vi "gateway发消息.vi"() -> ()   [LabVIEW 2012]
uses:
  <vilib>/LabVIEW Targets/Embedded/WSN/Host API/WSN Msg Status.ctl
panel:
  out "message status":T1
  in  "停止":bool
  in  "更改":bool
  in  "取消按钮":bool
  out "节点信息":string
  in  "节点":i32(listbox)
  in  "确定按钮":bool
  out "返回消息":string
  in  "发消息":string
  in  "网关IP地址":string
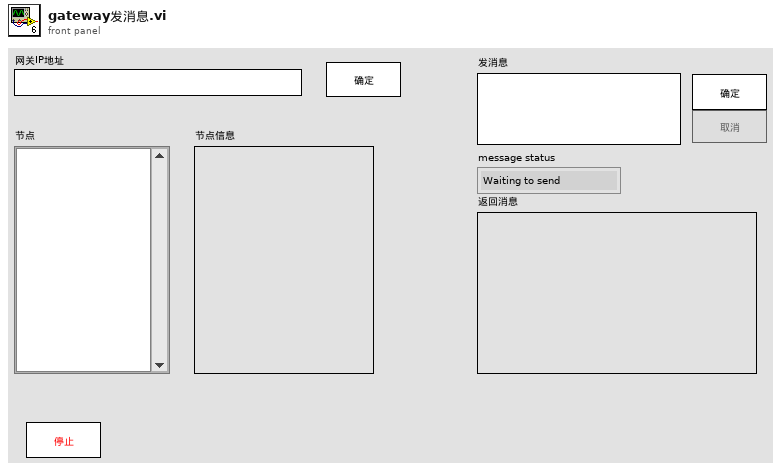
[diagram p1: front panel]
types:
  T1 = typedef "WSN Msg Status.ctl" = enum8{"Waiting to send", "Sent to node", "Failed", "Cancelled"}
  T2 = enum8{"Enabled", "Disabled", "Disabled and Grayed Out"}
  T3 = typedef "WSN Node Info.ctl" = cluster{"Serial Number":u32, "ID":u32, "Node Type":u16, "Firmware Update State":enum8{"Not Started", "In Progress", "Error", "Done"}, "Firmware Update Percent Complete":u8, "Current Firmware Version":string, "Battery State":u8, "Last Packet Received":timestamp, "Link Quality":enum16{"No Signal", "Poor", "Fair", "Good", "Excellent"}, "Power Supply":enum8{"Battery", "Externally Powered"}, "Network Mode":enum8{"End Device", "Mesh Router"}}
  T4 = typedef "WSN Message.ctl" = cluster{"Message Type":enum16{"User Message", "Debug Message"}, "Message Timestamp":timestamp, "Data":string}
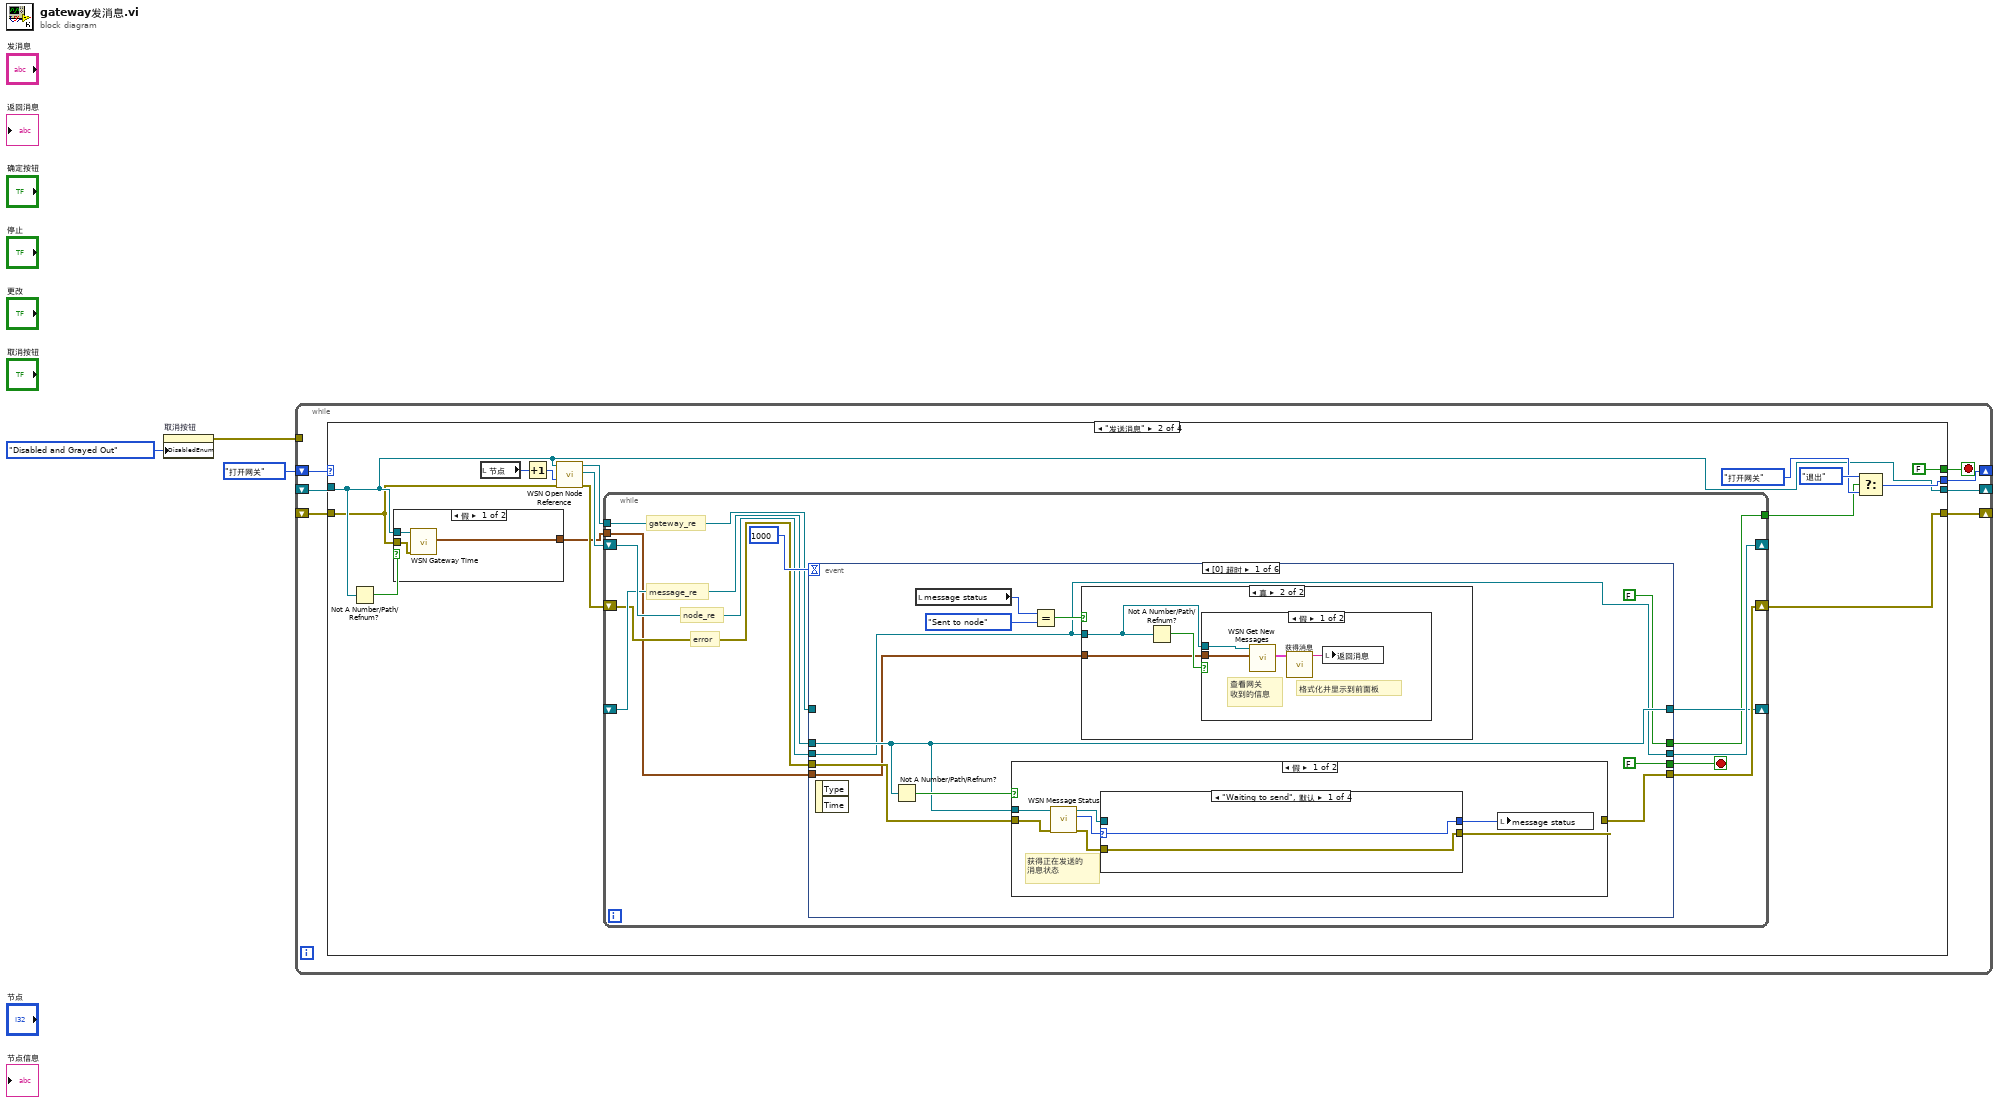
[diagram p0: block diagram]
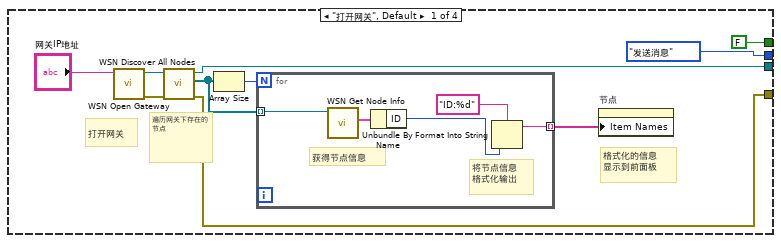
[diagram p2: hidden frame]
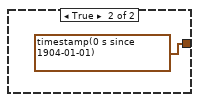
[diagram p3: hidden frame]
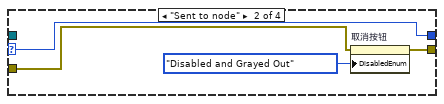
[diagram p6: hidden frame]
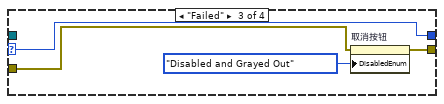
[diagram p7: hidden frame]
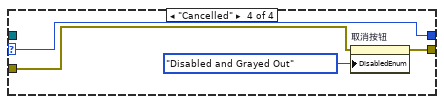
[diagram p8: hidden frame]
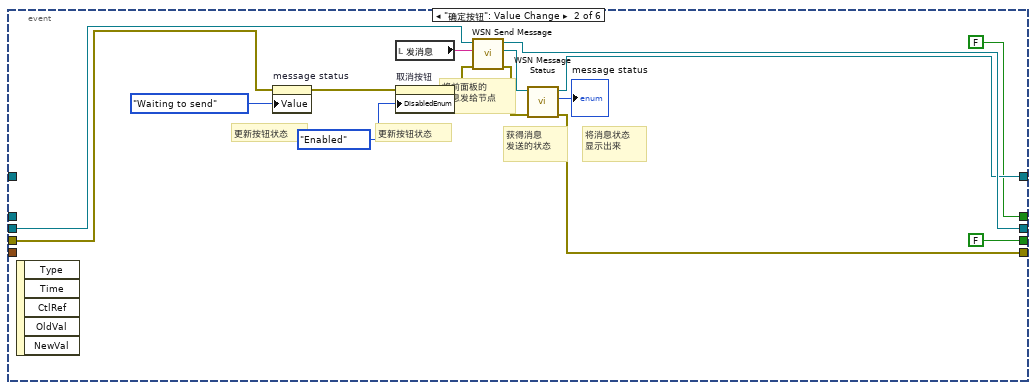
[diagram p10: hidden frame]
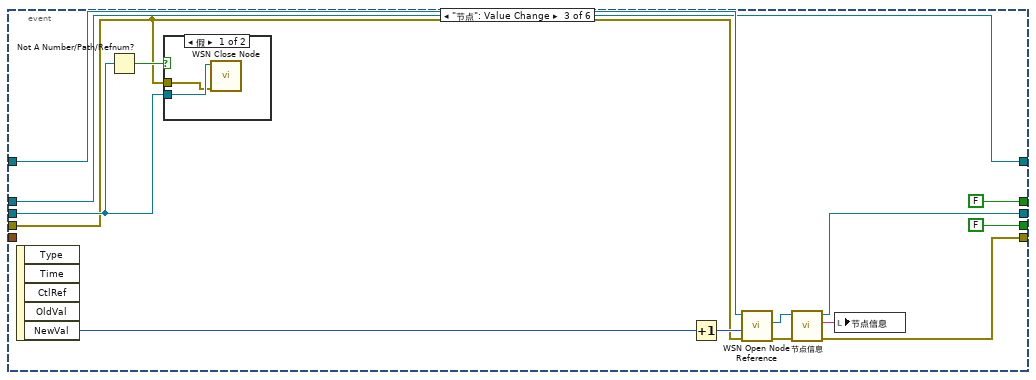
[diagram p11: hidden frame]
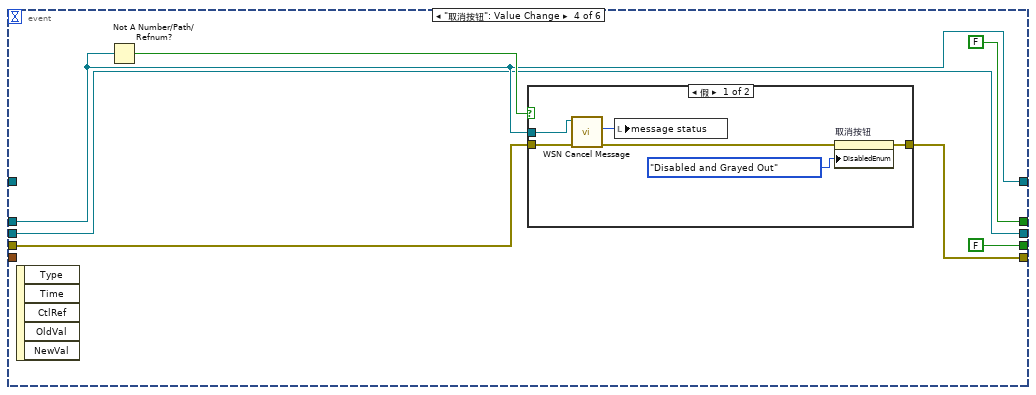
[diagram p13: hidden frame]
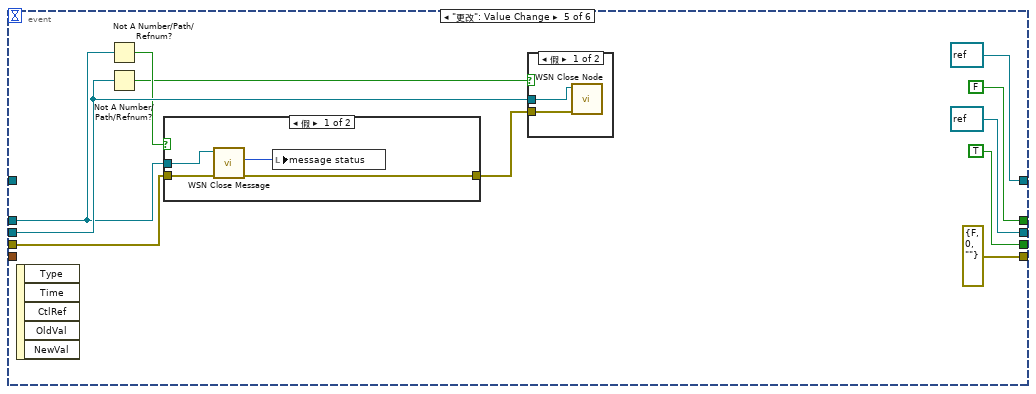
[diagram p15: hidden frame]
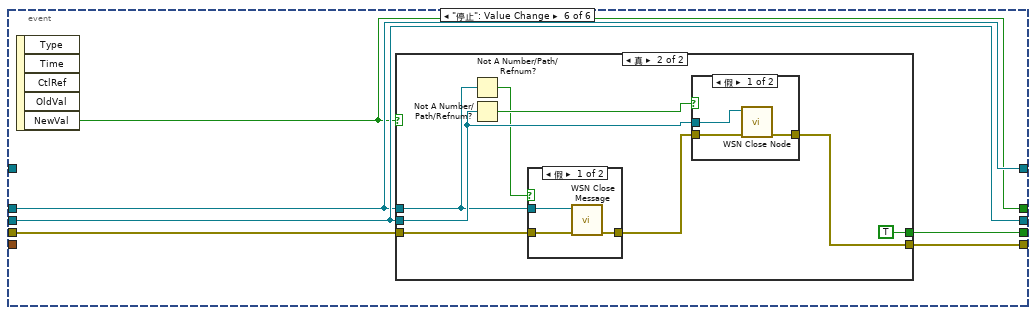
[diagram p18: hidden frame]
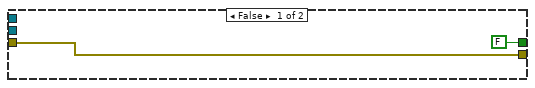
[diagram p19: hidden frame]
diagram:
  n1 = property on="取消按钮" class="Bool"("DisabledEnum"=T2."Disabled and Grayed Out" ("禁用")) -> (error out=w1:errorcluster)  [unwired: 2 in, 1 out]
  n2 = while {
    shift-right: [w4] -> _
    shift-left: enum16{"打开网关", "发送消息", "关闭网关", "退出"}."打开网关" -> [w10]
    shift-right: [w9] -> _
    shift-left: _ -> [w7]
    shift-right: [w8] -> _
    shift-left: _ -> [w6]
    tunnel: w1 -> [_]
    stop <- w5 stop-if-true
    n3 = case shown="\"发送消息\"" w10 {
      tunnel: [w14 w28 w184 refnum<k20> refnum ("gateway reference")] -> w9
      tunnel: [w13 w37 errorcluster {"status"=FALSE, "code"=0, "source"=""} ("error out") errorcluster {"status"=FALSE, "code"=0, "source"=""} ("error out")] -> w8
      tunnel: w7 -> [_ w28 w184 w192]
      tunnel: w6 -> [_ w27 w188 w196]
      tunnel: [FALSE FALSE FALSE TRUE] -> w5
      tunnel: [enum16{"打开网关", "发送消息", "关闭网关", "退出"}."发送消息" w35 enum16{"打开网关", "发送消息", "关闭网关", "退出"}."打开网关" enum16{"打开网关", "发送消息", "关闭网关", "退出"}."打开网关"] -> w4
      frame "打开网关", Default {
        # "格式化的信息\n显示到前面板"
        # "遍历网关下存在的节点"
        # "打开网关"
        n4 = call <vilib>:"WSN Open Gateway.vi"("IP address"="网关IP地址") -> ("error out"=w18:errorcluster, "gateway reference"=w19:refnum<k20>)  [unwired: 9 in]
        n5 = call <vilib>:"WSN Discover All Nodes.vi"("error in (no error)"=w18, "gateway reference"=w19) -> ("error out"=w13:errorcluster, "node references"=w16:refnum<k20>[], "gateway reference"=w14:refnum<k20>)  [unwired: 7 in]
        n6 = Array Size(array=w16) -> (size(s)=w17:i32)
        n7 = for {
          N: w17 -> [_]
          tunnel: w16 -> [w25] mode=indexing
          tunnel: [w22] -> w15 mode=indexing
          # "获得节点信息"
          # "将节点信息\n格式化输出"
          n8 = call <vilib>:"WSN Get Node Info.vi"("node reference"=w25) -> ("node information"=w24:T3)  [unwired: 8 in, 2 out]
          n9 = Unbundle By Name(w24) -> ("ID"=w21:u32)
          n10 = Format Into String(format string="ID:%d" ("格式字符串"), w21) -> (resulting string=w22:string)  [unwired: 2 in, 1 out]
        }
        n11 = property on="节点" class="LstBox (严格)"("Item Names"=w15) -> ()  [unwired: 2 in, 2 out]
      }
      frame "发送消息" {
        n12 = Not A Number/Path/Refnum?(number/path/refnum=w28) -> (NaN/Path/Refnum?=w29:bool)
        n13 = case shown="假" w29 {
          tunnel: w28 -> [w43 _]
          tunnel: w27 -> [w42 _]
          tunnel: [w41 timestamp(0 s since 1904-01-01) ("time")] -> w26
          frame False {
            n14 = call <vilib>:"WSN Gateway Time.vi"("error in (no error)"=w42, "gateway reference"=w43) -> ("time"=w41:timestamp)  [unwired: 7 in, 2 out]
          }
          frame True {
          }
        }
        n15 = local read "节点"() -> (w31:i32)
        n16 = Increment(x=w31) -> (x+1=w30:i32)
        n17 = call <vilib>:"WSN Open Node Reference.vi"("error in (no error)"=w27, "ID"=w30, "gateway reference"=w28) -> ("error out"=w39:errorcluster, "node reference"=w40:refnum<k20>, "gateway reference"=w38:refnum<k20>)  [unwired: 6 in]
        n18 = while {
          shift-right: [w53] -> _
          shift-left: w40 -> [w52]
          shift-right: [w54] -> w37
          shift-left: w39 -> [w46]
          tunnel: w38 -> [w47]
          shift-right: [w51] -> _
          shift-left: _ -> [w50]
          tunnel: [w48] -> w32
          tunnel: w26 -> [w45]
          stop <- w49 stop-if-true
          # "gateway_re"
          # "message_re"
          # "error"
          # "node_re"
          n19 = event shown="[0] 超时" {
            selector: _ -> [_ _ _ _ _ _]
            dyn-events: _ -> [_ _ _ _ _ _]
            timeout: 1000 -> [_ _ _ _ _ _]
            tunnel: [w64 w106 w115 w130 errorcluster {"status"=FALSE, "code"=0, "source"=""} ("error out") w162] -> w54
            tunnel: [w58 w107 w116 w129 refnum<k20> refnum ("node reference") w161] -> w53
            tunnel: w52 -> [w58 w110 w120 w129 w144 w161]
            tunnel: w46 -> [w61 w97 w111 w132 w150 w163]
            tunnel: w47 -> [_ _ w124 _ _ _]
            tunnel: [w65 w103 w123 w131 refnum<k20> refnum ("message reference") w160] -> w51
            tunnel: w50 -> [w65 _ w123 w131 w143 w160]
            tunnel: [FALSE FALSE FALSE FALSE TRUE w164] -> w49
            tunnel: [FALSE ("NewVal") FALSE ("NewVal") FALSE ("NewVal") FALSE ("NewVal") FALSE ("NewVal") w159] -> w48
            tunnel: w45 -> [w57 _ _ _ _ _]
            event Timeout {
              n20 = event-data() -> ()  [unwired: 1 in, 2 out]
              n21 = Not A Number/Path/Refnum?(number/path/refnum=w65) -> (NaN/Path/Refnum?=w66:bool)
              n22 = local read "message status"() -> (w56:T1)
              n23 = case shown="假" w66 {
                tunnel: [w80 w95] -> w64
                tunnel: w61 -> [w78 w95]
                tunnel: w65 -> [w75 _]
                frame False {
                  # "获得正在发送的\n消息状态"
                  n24 = call <vilib>:"WSN Message Status.vi"("error in (no error)"=w78, "message reference"=w75) -> ("error out"=w77:errorcluster, "message status"=w76:T1, "message reference"=w79:refnum<k20>)  [unwired: 7 out]
                  n25 = case shown="\"Waiting to send\", 默认" w76 {
                    selector: w76 -> [w81 w86 w90 w94]
                    tunnel: w79 -> [_ _ _ _]
                    tunnel: w77 -> [w82 w85 w89 w93]
                    tunnel: [w82 w84 w88 w92] -> w80
                    tunnel: [w81 w86 w90 w94] -> w74
                    frame "Waiting to send", Default {
                    }
                    frame "Sent to node" {
                      n26 = property on="取消按钮" class="Bool"(error in=w85, "DisabledEnum"=T2."Disabled and Grayed Out" ("禁用")) -> (error out=w84:errorcluster)  [unwired: 1 in, 1 out]
                    }
                    frame "Failed" {
                      n27 = property on="取消按钮" class="Bool"(error in=w89, "DisabledEnum"=T2."Disabled and Grayed Out" ("禁用")) -> (error out=w88:errorcluster)  [unwired: 1 in, 1 out]
                    }
                    frame "Cancelled" {
                      n28 = property on="取消按钮" class="Bool"(error in=w93, "DisabledEnum"=T2."Disabled and Grayed Out" ("禁用")) -> (error out=w92:errorcluster)  [unwired: 1 in, 1 out]
                    }
                  }
                  n29 = local write "message status"(w74) -> ()
                }
                frame True {
                }
              }
              n30 = Equal?(x=w56, y=WSN_Msg_Status."Sent to node" ("x")) -> (x = y?=w59:bool)
              n31 = case shown="真" w59 {
                tunnel: w58 -> [_ w68]
                tunnel: w57 -> [_ w67]
                frame False {
                }
                frame True {
                  n32 = Not A Number/Path/Refnum?(number/path/refnum=w68) -> (NaN/Path/Refnum?=w69:bool)
                  n33 = case shown="假" w69 {
                    tunnel: w68 -> [w73 _]
                    tunnel: w67 -> [w72 _]
                    frame False {
                      # "格式化并显示到前面板"
                      # "查看网关\n收到的信息"
                      n34 = call <vilib>:"WSN Get New Messages.vi"("starting time"=w72, "node reference"=w73) -> ("messages"=w71:T4[])  [unwired: 7 in, 2 out]
                      n35 = call "获得消息.vi"("messages"=w71) -> ("连接的字符串"=w70:string)  [unwired: 10 in]
                      n36 = local write "返回消息"(w70) -> ()
                    }
                    frame True {
                    }
                  }
                }
              }
            }
            event "确定按钮": Value Change {
              # "更新按钮状态"
              # "更新按钮状态"
              # "将消息状态\n显示出来"
              # "获得消息\n发送的状态"
              # "将前面板的\n消息发给节点"
              n37 = event-data() -> ()  [unwired: 1 in, 5 out]
              n38 = property on="message status" class="Enum (严格)"(error in=w97, "Value"=WSN_Msg_Status."Waiting to send" ("message status")) -> (error out=w96:errorcluster)  [unwired: 1 in, 1 out]
              n39 = local read "发消息"() -> (w109:string)
              n40 = property on="取消按钮" class="Bool"(error in=w96, "DisabledEnum"=T2."Enabled" ("禁用")) -> (error out=w104:errorcluster)  [unwired: 1 in, 1 out]
              n41 = call <vilib>:"WSN Send Message.vi"("error in (no error)"=w104, "message"=w109, "node reference"=w110) -> ("error out"=w100:errorcluster, "message reference"=w108:refnum<k20>, "node reference"=w107:refnum<k20>)  [unwired: 6 in]
              n42 = call <vilib>:"WSN Message Status.vi"("error in (no error)"=w100, "message reference"=w108) -> ("error out"=w106:errorcluster, "message status"=→"message status":T1, "message reference"=w103:refnum<k20>)  [unwired: 7 in]
            }
            event "节点": Value Change {
              n43 = event-data() -> ("NewVal"=w113:i32)  [unwired: 1 in, 4 out]
              n44 = Not A Number/Path/Refnum?(number/path/refnum=w120) -> (NaN/Path/Refnum?=w121:bool)
              n45 = case shown="假" w121 {
                tunnel: w120 -> [w126 _]
                tunnel: w111 -> [w125 _]
                frame False {
                  n46 = call <vilib>:"WSN Close Node.vi"("error in (no error)"=w125, "node reference"=w126) -> ()  [unwired: 9 in, 1 out]
                }
                frame True {
                }
              }
              n47 = Increment(x=w113) -> (x+1=w112:i32)
              n48 = call <vilib>:"WSN Open Node Reference.vi"("error in (no error)"=w111, "ID"=w112, "gateway reference"=w124) -> ("error out"=w118:errorcluster, "node reference"=w119:refnum<k20>)  [unwired: 6 in, 1 out]
              n49 = call "节点信息.vi"("node reference"=w119, "error in (no error)"=w118) -> ("node reference 2"=w116:refnum<k20>, "连接的字符串"=w117:string, "error out"=w115:errorcluster)  [unwired: 6 in]
              n50 = local write "节点信息"(w117) -> ()
            }
            event "取消按钮": Value Change {
              n51 = event-data() -> ()  [unwired: 1 in, 5 out]
              n52 = Not A Number/Path/Refnum?(number/path/refnum=w131) -> (NaN/Path/Refnum?=w133:bool)
              n53 = case shown="假" w133 {
                tunnel: w131 -> [w139 _]
                tunnel: w132 -> [w138 w140]
                tunnel: [w135 w140] -> w130
                frame False {
                  n54 = call <vilib>:"WSN Cancel Message.vi"("error in (no error)"=w138, "message reference"=w139) -> ("error out"=w136:errorcluster, "message status"=w134:T1)  [unwired: 7 in, 1 out]
                  n55 = local write "message status"(w134) -> ()
                  n56 = property on="取消按钮" class="Bool"(error in=w136, "DisabledEnum"=T2."Disabled and Grayed Out" ("禁用")) -> (error out=w135:errorcluster)  [unwired: 1 in, 1 out]
                }
                frame True {
                }
              }
            }
            event "更改": Value Change {
              n57 = event-data() -> ()  [unwired: 1 in, 5 out]
              n58 = Not A Number/Path/Refnum?(number/path/refnum=w143) -> (NaN/Path/Refnum?=w142:bool)
              n59 = Not A Number/Path/Refnum?(number/path/refnum=w144) -> (NaN/Path/Refnum?=w141:bool)
              n60 = case shown="假" w142 {
                tunnel: w150 -> [w157 w158]
                tunnel: [w156 w158] -> w149
                tunnel: w143 -> [w155 _]
                frame False {
                  n61 = call <vilib>:"WSN Close Message.vi"("error in (no error)"=w157, "message reference"=w155) -> ("error out"=w156:errorcluster, "message status"=w154:T1)  [unwired: 8 in]
                  n62 = local write "message status"(w154) -> ()
                }
                frame True {
                }
              }
              n63 = case shown="假" w141 {
                tunnel: w149 -> [w153 _]
                tunnel: w144 -> [w152 _]
                frame False {
                  n64 = call <vilib>:"WSN Close Node.vi"("error in (no error)"=w153, "node reference"=w152) -> ()  [unwired: 9 in, 1 out]
                }
                frame True {
                }
              }
            }
            event "停止": Value Change {
              n65 = event-data() -> ("NewVal"=w159:bool)  [unwired: 1 in, 4 out]
              n66 = case shown="真" w159 {
                tunnel: [FALSE TRUE] -> w164
                tunnel: w161 -> [_ w172]
                tunnel: w163 -> [w165 w169]
                tunnel: w160 -> [_ w170]
                tunnel: [w165 w167] -> w162
                frame False {
                }
                frame True {
                  n67 = Not A Number/Path/Refnum?(number/path/refnum=w170) -> (NaN/Path/Refnum?=w171:bool)
                  n68 = Not A Number/Path/Refnum?(number/path/refnum=w172) -> (NaN/Path/Refnum?=w173:bool)
                  n69 = case shown="假" w171 {
                    tunnel: w170 -> [w177 _]
                    tunnel: w169 -> [w176 w178]
                    tunnel: [w175 w178] -> w168
                    frame False {
                      n70 = call <vilib>:"WSN Close Message.vi"("error in (no error)"=w176, "message reference"=w177) -> ("error out"=w175:errorcluster)  [unwired: 8 in, 1 out]
                    }
                    frame True {
                    }
                  }
                  n71 = case shown="假" w173 {
                    tunnel: w172 -> [w181 _]
                    tunnel: w168 -> [w180 w182]
                    tunnel: [w179 w182] -> w167
                    frame False {
                      n72 = call <vilib>:"WSN Close Node.vi"("error in (no error)"=w180, "node reference"=w181) -> ("error out"=w179:errorcluster)  [unwired: 9 in]
                    }
                    frame True {
                    }
                  }
                }
              }
            }
          }
        }
        n73 = Select(t=enum16{"打开网关", "发送消息", "关闭网关", "退出"}."退出", s=w32, f=enum16{"打开网关", "发送消息", "关闭网关", "退出"}."打开网关") -> (s? t:f=w35:enum16{"打开网关", "发送消息", "关闭网关", "退出"})
      }
      frame "关闭网关" {
        n74 = Not A Number/Path/Refnum?(number/path/refnum=w184) -> (NaN/Path/Refnum?=w183:bool)
        n75 = case shown="假" w183 {
          tunnel: w188 -> [w190 _]
          tunnel: w184 -> [w189 _]
          frame False {
            n76 = call <vilib>:"WSN Close Gateway.vi"("error in (no error)"=w190, "gateway reference"=w189) -> ()  [unwired: 9 in, 1 out]
          }
          frame True {
          }
        }
      }
      frame "退出" {
        n77 = Not A Number/Path/Refnum?(number/path/refnum=w192) -> (NaN/Path/Refnum?=w191:bool)
        n78 = case shown="假" w191 {
          tunnel: w196 -> [w199 _]
          tunnel: w192 -> [w198 _]
          frame False {
            n79 = call <vilib>:"WSN Close Gateway.vi"("error in (no error)"=w199, "gateway reference"=w198) -> ()  [unwired: 9 in, 1 out]
          }
          frame True {
          }
        }
      }
    }
  }
